vi "Append Text Table to Report.vi"(0 "report in":refnum<class "ooWriter.lvclass">, 1 "column width (1)":dbl=1.0 format="%.2f", 2 "measurement system":u16(ring)=2 caption="measurement system for column width (Default)" items=["US", "Metric", "Default"], 3 "MS Office parameters":T2, 5 "column headers":string[](array[string]), 7 "row headers":string[](array[string]), 9 "text data":string[][](array[string]), 11 "error in (no error)":errorcluster, 13 "separate page?":bool, 14 "show grid lines":bool=TRUE) -> (4 "report out":refnum<class "ooWriter.lvclass">, 8 "range (wd) - start (xl)":T1, 10 "end (xl)":cluster{"row (xl) ":i32, "col (xl) ":i32}, 15 "error out":errorcluster)   [LabVIEW 2009, in "ooWriter.lvclass"]
doc: "Appends a 2D array to a report as a table with the given column width. You can use this polymorphic VI to append an array of strings or numbers. The data type you wire to the <B>text data</B> input determines the polymorphic instance to use."
uses:
  ooWriter.lvclass
  ooWriter.lvclass/ooWriter.ctl
  C:/Projets/LAVAG/OpenOfficeRGT/AODL/DLLs/AODL.dll
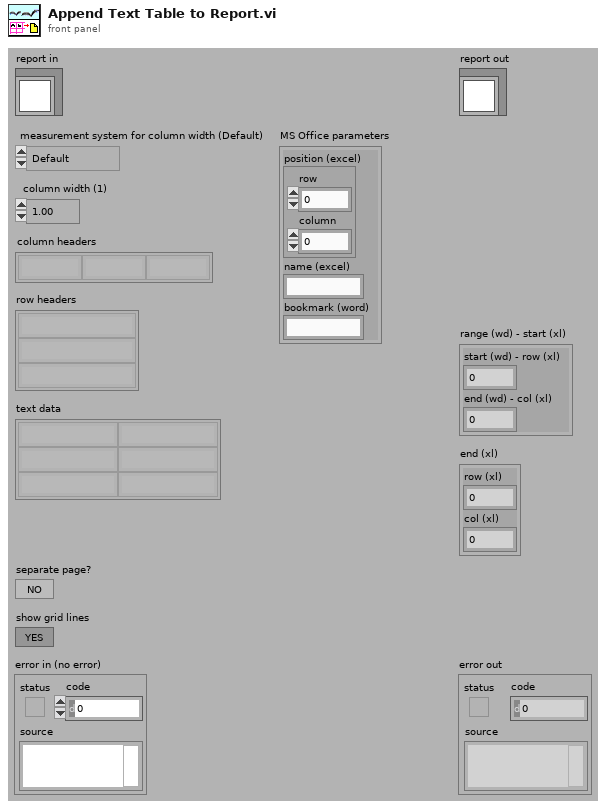
[diagram p1: front panel]
types:
  T1 = cluster{"start (wd) - row (xl) ":i32, "end (wd) - col (xl) ":i32}
  T2 = cluster{"position (excel)":cluster{"row":i32, "column":i32}, "name (excel)":string, "bookmark (word)":string}
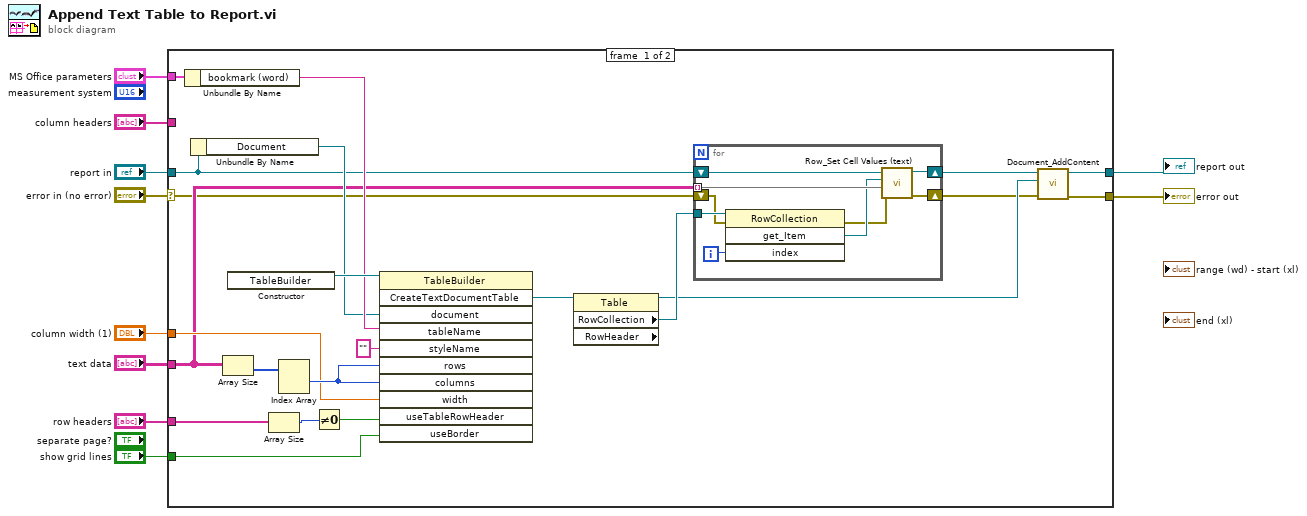
[diagram p0: block diagram]
diagram:
  n1 = case shown="No Error" "error in (no error)" {
    selector: "error in (no error)" -> [w11 w42]
    tunnel: [w18 w42] -> w9
    tunnel: "report in" -> [w17 w43]
    tunnel: [w19 w43] -> w7
    tunnel: "show grid lines" -> [w29 _]
    tunnel: "text data" -> [w15 _]
    tunnel: "column width (1)" -> [w26 _]
    tunnel: "MS Office parameters" -> [w25 _]
    tunnel: "column headers" -> [_ _]
    tunnel: "row headers" -> [w22 _]
    frame #0 {
      n2 = Unbundle By Name(w25) -> ("bookmark (word)"=w24:string)
      n3 = Unbundle By Name(w17) -> ("Document"=w21:refnum<k24>)
      n4 = Array Size(array=w15) -> (size(s)=w28:i32[])
      n5 = constructor class="TableBuilder"() -> (reference out=w32:refnum<k24>)  [unwired: 3 in, 2 out]
      n6 = Array Size(array=w22) -> (size(s)=w31:i32)
      n7 = Index Array(array=w28) -> (element #1=w27:i32)  [unwired: 2 in, 1 out]
      n8 = Not Equal To 0?(x=w31) -> (x != 0?=w30:bool)
      n9 = invoke class="TableBuilder" method="CreateTextDocumentTable"(reference=w32, "document"=w21, "tableName"=w24, "styleName"="", "rows"=w27, "columns"=w27, "width"=w26, "useTableRowHeader"=w30, "useBorder"=w29) -> ("CreateTextDocumentTable"=w20:refnum<k24>)  [unwired: 2 in, 10 out]
      n10 = property class="Table" props=["RowCollection", "RowHeader"](reference=w20) -> (reference out=w13:refnum<k24>, "RowCollection"=w14:refnum<k24>)  [unwired: 1 in, 2 out]
      n11 = for {
        shift-right: [w40] -> w16
        shift-left: w17 -> [w41]
        tunnel: w15 -> [w39] mode=indexing
        tunnel: w14 -> [w37]
        shift-right: [w34] -> w12
        shift-left: w11 -> [w33]
        i -> [w38]
        n12 = invoke class="RowCollection" method="get_Item"(reference=w37, error in=w33, "index"=w38) -> (error out=w35:errorcluster, "get_Item"=w36:refnum<k24>)  [unwired: 1 in, 2 out]
        n13 = call-dynamic "Row_Set Cell Values (text).vi"("error in (no error)"=w35, "text data (row)"=w39, "Row"=w36, "ooWriter in"=w41) -> ("error out"=w34:errorcluster, "ooWriter out"=w40:refnum<class "ooWriter.lvclass">)  [unwired: 6 in]
      }
      n14 = call-dynamic "Document_AddContent.vi"("error in (no error)"=w12, "Content"=w13, "ooWriter in"=w16) -> ("error out"=w18:errorcluster, "ooWriter out"=w19:refnum<class "ooWriter.lvclass">)  [unwired: 7 in]
    }
    frame #1 {
    }
  }
  "error out" <- w9
  "report out" <- w7
